vi "Set Security Level.vi"(8 "error in (no error)":errorcluster, 10 "New Level":T1, 11 "Security System in":refnum<class "Security System.lvclass">) -> (0 "error out":errorcluster, 2 "Last Action Performed":string, 3 "Security System out":refnum<class "Security System.lvclass">)   [LabVIEW 2020, in "Security System.lvclass"]
uses:
  Security System.lvclass
  Security Level.ctl
  Set or Clear.ctl
  Security System.lvclass/Security System.ctl
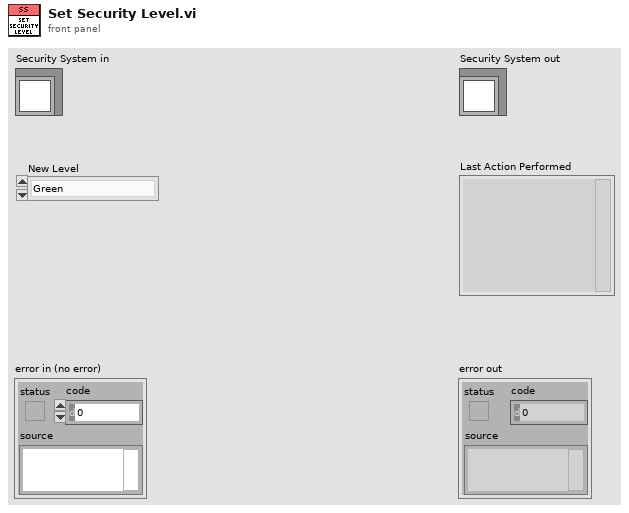
[diagram p1: front panel]
types:
  T1 = typedef "Security System.lvclass/Security Level.ctl" = enum16{"Green", "Yellow", "Orange", "Red"}
  T2 = typedef "Security System.lvclass/Set or Clear.ctl" = enum16{"Set", "Clear"}
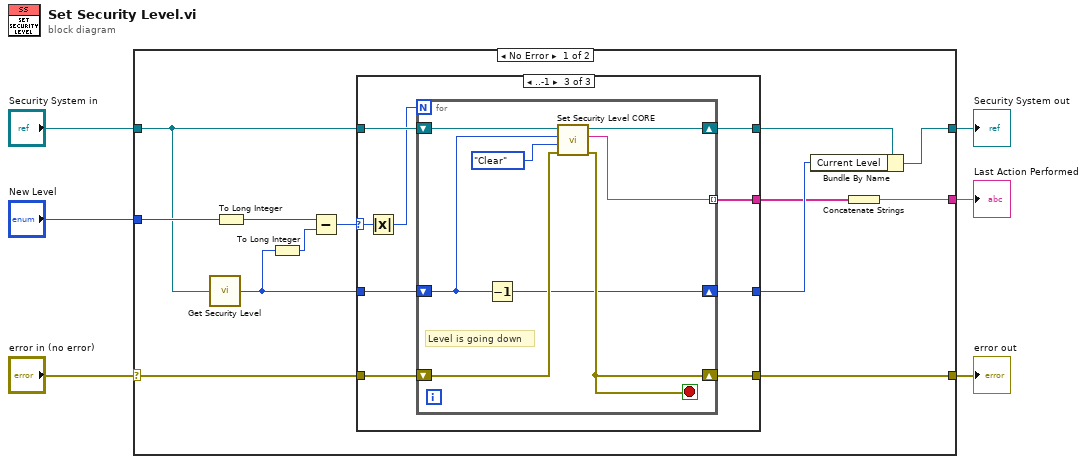
[diagram p0: block diagram]
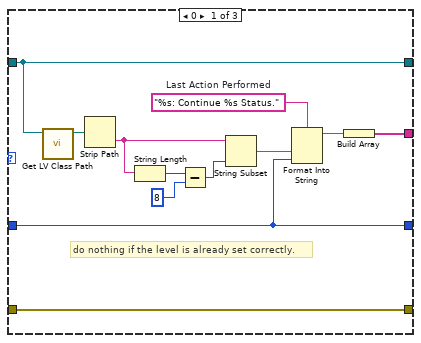
[diagram p2: hidden frame]
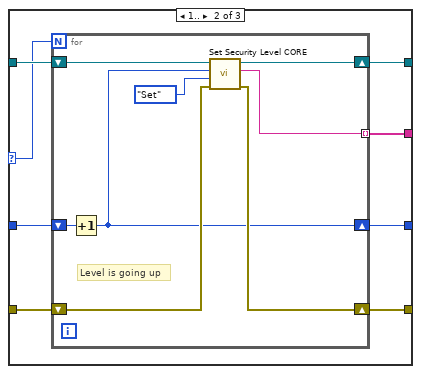
[diagram p3: hidden frame]
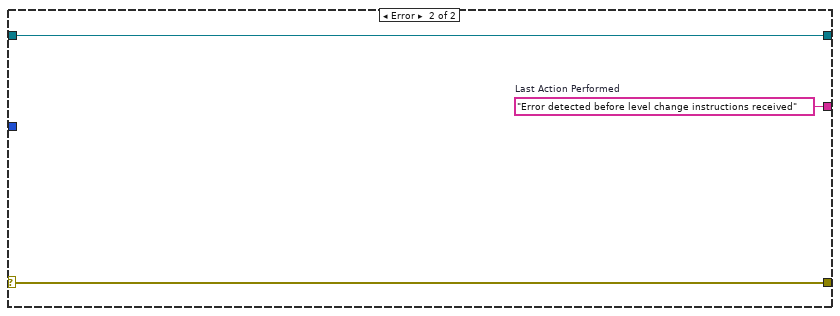
[diagram p4: hidden frame]
diagram:
  n1 = case shown="No Error" "error in (no error)" {
    selector: "error in (no error)" -> [w15 w67]
    tunnel: [w13 w67] -> w5
    tunnel: [w10 w66] -> w3
    tunnel: "Security System in" -> [w14 w66]
    tunnel: "New Level" -> [w19 _]
    tunnel: [w7 w65] -> w1
    frame No Error {
      n2 = call "Get Security Level.vi"("Security System.lvclass"=w14) -> ("Current Level"=w12:T1)
      n3 = To Long Integer(number=w19) -> (32bit integer=w18:i32)
      n4 = To Long Integer(number=w12) -> (32bit integer=w17:i32)
      n5 = Subtract(x=w18, y=w17) -> (x-y=w16:i32)
      n6 = case shown="..-1" w16 {
        selector: w16 -> [_ w36 w53]
        tunnel: w15 -> [w31 w37 w54]
        tunnel: w14 -> [w30 w39 w56]
        tunnel: [w30 w38 w55] -> w11
        tunnel: [w31 w35 w52] -> w13
        tunnel: w12 -> [w20 w34 w51]
        tunnel: [w21 w32 w49] -> w8
        tunnel: [w20 w33 w50] -> w9
        frame 0 {
          w24 = "%s: Continue %s Status."  # Last Action Performed
          # "do nothing if the level is already set correctly."
          n7 = call <vilib>:"Get LV Class Path.vi"("object"=w30) -> ("class path"=w29:path)  [unwired: 9 in, 1 out]
          n8 = Strip Path(path=w29) -> (name=w28:string)  [unwired: 1 out]
          n9 = String Length(string=w28) -> (length=w27:i32)
          n10 = Subtract(x=w27, y=8) -> (x-y=w25:i32)
          n11 = String Subset(string=w28, length (rest)=w25) -> (substring=w23:string)  [unwired: 1 in]
          n12 = Format Into String(format string=w24, w23, w20) -> (resulting string=w22:string)  [unwired: 2 in, 1 out]
          n13 = Build Array(w22) -> (w21:string[])
        }
        frame 1.. {
          n14 = for {
            N: w36 -> [_]
            shift-right: [w46] -> w38
            shift-left: w39 -> [w47]
            shift-right: [w44] -> w35
            shift-left: w37 -> [w45]
            shift-right: [w42] -> w33
            shift-left: w34 -> [w43]
            tunnel: [w40] -> w32 mode=indexing
            # "Level is going up"
            n15 = Increment(x=w43) -> (x+1=w42:T1)
            n16 = call-dynamic "Set Security Level CORE.vi"("error in (no error)"=w45, "Set or Clear"=Set_or_Clear."Set", "Security Level"=w42, "Security System in"=w47) -> ("error out"=w44:errorcluster, "Last Action Performed"=w40:string, "Security System out"=w46:refnum<class "Security System.lvclass">)  [unwired: 5 in]
          }
        }
        frame ..-1 {
          n17 = Absolute Value(x=w53) -> (abs(x)=w48:i32)
          n18 = for {
            N: w48 -> [_]
            shift-right: [w63] -> w55
            shift-left: w56 -> [w64]
            shift-right: [w59] -> w52
            shift-left: w54 -> [w62]
            shift-right: [w57] -> w50
            shift-left: w51 -> [w58]
            tunnel: [w60] -> w49 mode=indexing
            stop <- w59 stop-if-true
            # "Level is going down"
            n19 = Decrement(x=w58) -> (x-1=w57:T1)
            n20 = call-dynamic "Set Security Level CORE.vi"("error in (no error)"=w62, "Set or Clear"=Set_or_Clear."Clear", "Security Level"=w58, "Security System in"=w64) -> ("error out"=w59:errorcluster, "Last Action Performed"=w60:string, "Security System out"=w63:refnum<class "Security System.lvclass">)  [unwired: 5 in]
          }
        }
      }
      n21 = Bundle By Name(cluster=w11, "Current Level"=w9) -> (w10:refnum<class "Security System.lvclass">)
      n22 = Concatenate Strings(w8) -> (w7:string)
    }
    frame Error {
      w65 = "Error detected before level change instructions received"  # Last Action Performed
    }
  }
  "error out" <- w5
  "Security System out" <- w3
  "Last Action Performed" <- w1
